vi "Pieces Description.vi"() -> (0 "Pieces Description":T1)   [LabVIEW 2017]
uses:
  Controls/Pieces Description.ctl
  Controls/Piece Description.ctl
  Controls/Pieces Geometry Names.ctl
  Controls/Coordinates.ctl
  Controls/Rotation State.ctl
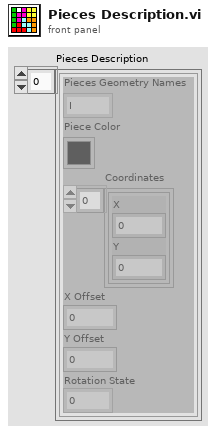
[diagram p1: front panel]
types:
  T1 = typedef "Pieces Description.ctl" = T2[]
  T2 = typedef "Piece Description.ctl" = cluster{"Pieces Geometry Names":T3, "Piece Color":u32, "Coordinates":T4[], "X Offset":i32, "Y Offset":i32, "Rotation State":T5}
  T3 = typedef "Pieces Geometry Names.ctl" = enum16{"I", "O", "T", "L", "J", "Z", "S"}
  T4 = typedef "Coordinates.ctl" = cluster{"X":i32, "Y":i32}
  T5 = typedef "Rotation State.ctl" = enum16{"0", "90", "180", "270"}
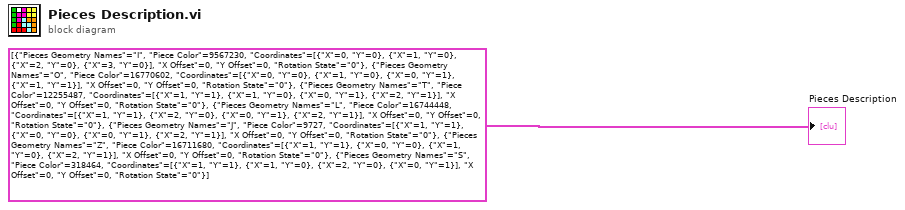
[diagram p0: block diagram]
diagram:
  "Pieces Description" <- T1 [{"Pieces Geometry Names"=enum."I", "Piece Color"=9567230, "Coordinates"=[{"X"=0, "Y"=0}, {"X"=1, "Y"=0}, {"X"=2, "Y"=0}, {"X"=3, "Y"=0}], "X Offset"=0, "Y Offset"=0, "Rotation State"=enum."0"}, {"Pieces Geometry Names"=enum."O", "Piece Color"=16770602, "Coordinates"=[{"X"=0, "Y"=0}, {"X"=1, "Y"=0}, {"X"=0, "Y"=1}, {"X"=1, "Y"=1}], "X Offset"=0, "Y Offset"=0, "Rotation State"=enum."0"}, {"Pieces Geometry Names"=enum."T", "Piece Color"=12255487, "Coordinates"=[{"X"=1, "Y"=1}, {"X"=1, "Y"=0}, {"X"=0, "Y"=1}, {"X"=2, "Y"=1}], "X Offset"=0, "Y Offset"=0, "Rotation State"=enum."0"}, {"Pieces Geometry Names"=enum."L", "Piece Color"=16744448, "Coordinates"=[{"X"=1, "Y"=1}, {"X"=2, "Y"=0}, {"X"=0, "Y"=1}, {"X"=2, "Y"=1}], "X Offset"=0, "Y Offset"=0, "Rotation State"=enum."0"}, {"Pieces Geometry Names"=enum."J", "Piece Color"=9727, "Coordinates"=[{"X"=1, "Y"=1}, {"X"=0, "Y"=0}, {"X"=0, "Y"=1}, {"X"=2, "Y"=1}], "X Offset"=0, "Y Offset"=0, "Rotation State"=enum."0"}, {"Pieces Geometry Names"=enum."Z", "Piece Color"=16711680, "Coordinates"=[{"X"=1, "Y"=1}, {"X"=0, "Y"=0}, {"X"=1, "Y"=0}, {"X"=2, "Y"=1}], "X Offset"=0, "Y Offset"=0, "Rotation State"=enum."0"}, {"Pieces Geometry Names"=enum."S", "Piece Color"=318464, "Coordinates"=[{"X"=1, "Y"=1}, {"X"=1, "Y"=0}, {"X"=2, "Y"=0}, {"X"=0, "Y"=1}], "X Offset"=0, "Y Offset"=0, "Rotation State"=enum."0"}] ("Pieces Description")
